vi "gfitsio-get-column-names.vi"(8 "error in (no error)":errorcluster, 11 "Refnum in":T1) -> (0 "error out":errorcluster, 2 "Array":string[](array[string]), 3 "Refnum out":T1)   [LabVIEW 2013]
uses:
  gfitsio-refnum.ctl
  gfitsio.lvlib
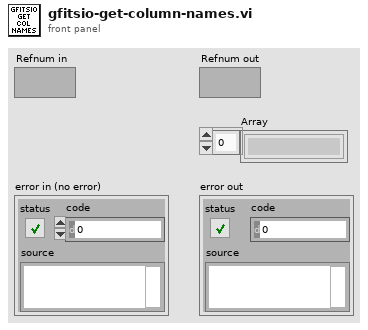
[diagram p1: front panel]
types:
  T1 = typedef "gfitsio.lvlib/gfitsio-refnum.ctl" = refnum<k1>
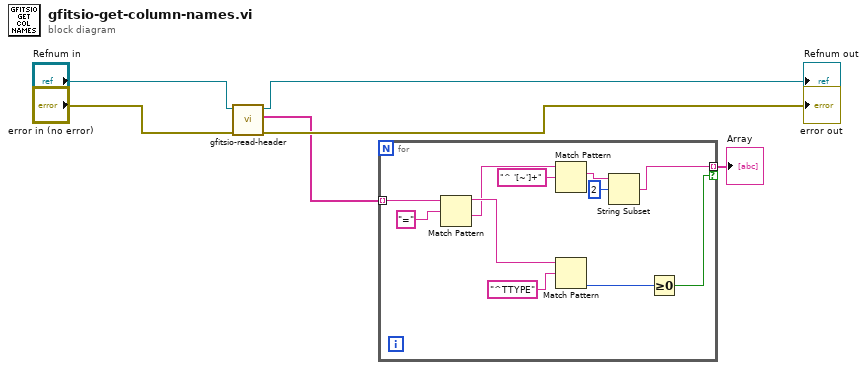
[diagram p0: block diagram]
diagram:
  n1 = call "gfitsio-read-header.vi"("error in (no error)"="error in (no error)", "gfits refnum"="Refnum in") -> ("error out"=→"error out":errorcluster, "header"=w3:string[], "dup gfits refnum"=→"Refnum out":T1)  [unwired: 7 in]
  n2 = for {
    tunnel: w3 -> [w17] mode=indexing
    tunnel: [w7] -> w4 mode=indexing if=w12
    n3 = Match Pattern(string=w17, regular expression="=") -> (before substring=w15:string, after substring=w10:string)  [unwired: 1 in, 2 out]
    n4 = Match Pattern(string=w10, regular expression="^ '[~']+") -> (match substring=w9:string)  [unwired: 1 in, 3 out]
    n5 = Match Pattern(string=w15, regular expression="^TTYPE") -> (offset past match=w13:i32)  [unwired: 1 in, 3 out]
    n6 = String Subset(string=w9, offset (0)=2) -> (substring=w7:string)  [unwired: 1 in]
    n7 = Greater Or Equal To 0?(x=w13) -> (x >= 0?=w12:bool)
  }
  "Array" <- w4
